vi "RT Loop - Analyze Acceleration_2.vi"(7 "testing":bool, 8 "error in (no error)":errorcluster, 9 "Acceleration RT FIFO In":T1, 10 "FPGA VI Reference Out":refnum<k20>, 11 "Message Queue":refnum<queue>) -> (1 "Acceleration RT FIFO Out":T1)   [LabVIEW 2017]
doc: "Read and analyze acceleration waveform data from FPGA via DMA FIFO. If the acceleration is over the limit, then send the acceleration waveform data to the Log Data Loop."
uses:
  UI Error Handlers/support/Message Queue/Message Cluster.ctl
  controls/Acceleration RT FIFO Reference.ctl
  Globals/Global - All RT Loop Stop.vi
  Globals/Global - Configuration Options.vi
  <vilib>/Utility/error.llb/Error Cluster From Error Code.vi
  <vilib>/rvi/errors/niLvFpgaAdjustHostInterfaceError.vi
  <vilib>/rvi/interface/nirviMethod/nirviMethod.xnode
  <vilib>/FPGAPlugInAG/Dynamic/niLvFpga_ReadFifo_Dynamic.vi
  <vilib>/rvi/errors/niLvFpgaMergeErrorWithErrorCode.vi
  UI Error Handlers/support/Logging/Logging.lvlib
  UI Error Handlers/support/Message Queue/Message Queue.lvlib
panel:
  out "G1 status":cluster{"G1 trigger":bool}
  out "G1 status.G1 trigger":bool
  out "sta":bool
  out "logical OR":bool
  in  "Data Rate (Hz)":dbl
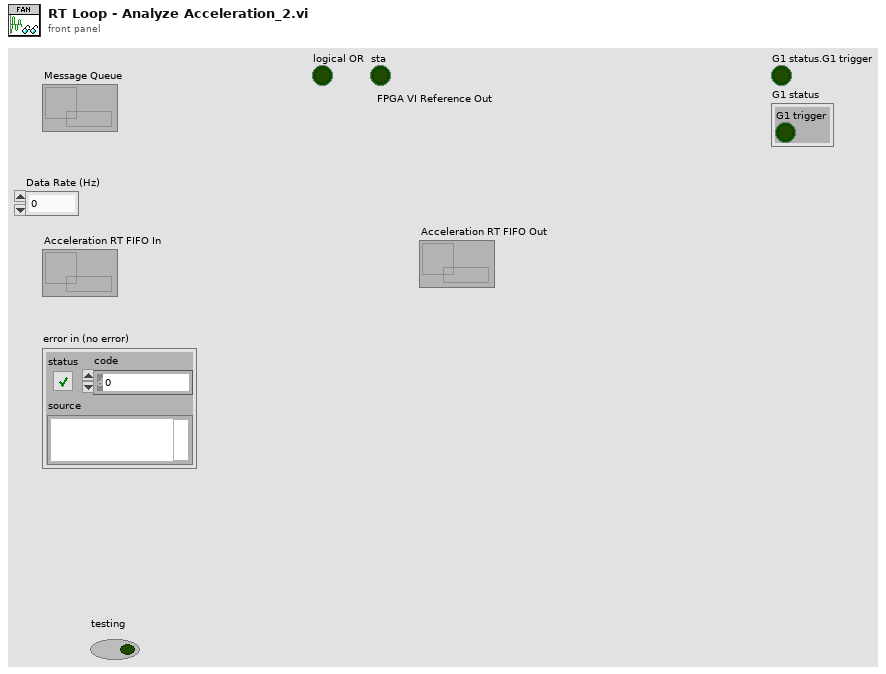
[diagram p1: front panel]
types:
  T1 = typedef "Acceleration RT FIFO Reference.ctl" = refnum<k33>
  T2 = cluster{"Tool data":cluster{"Number of teeth":sgl}, "Cutting data":cluster{"rpm":sgl}, "Limits":cluster{"Magnitude threshold":sgl, "Tolerance":sgl}, "G1 status":cluster{"G1 trigger":bool}}
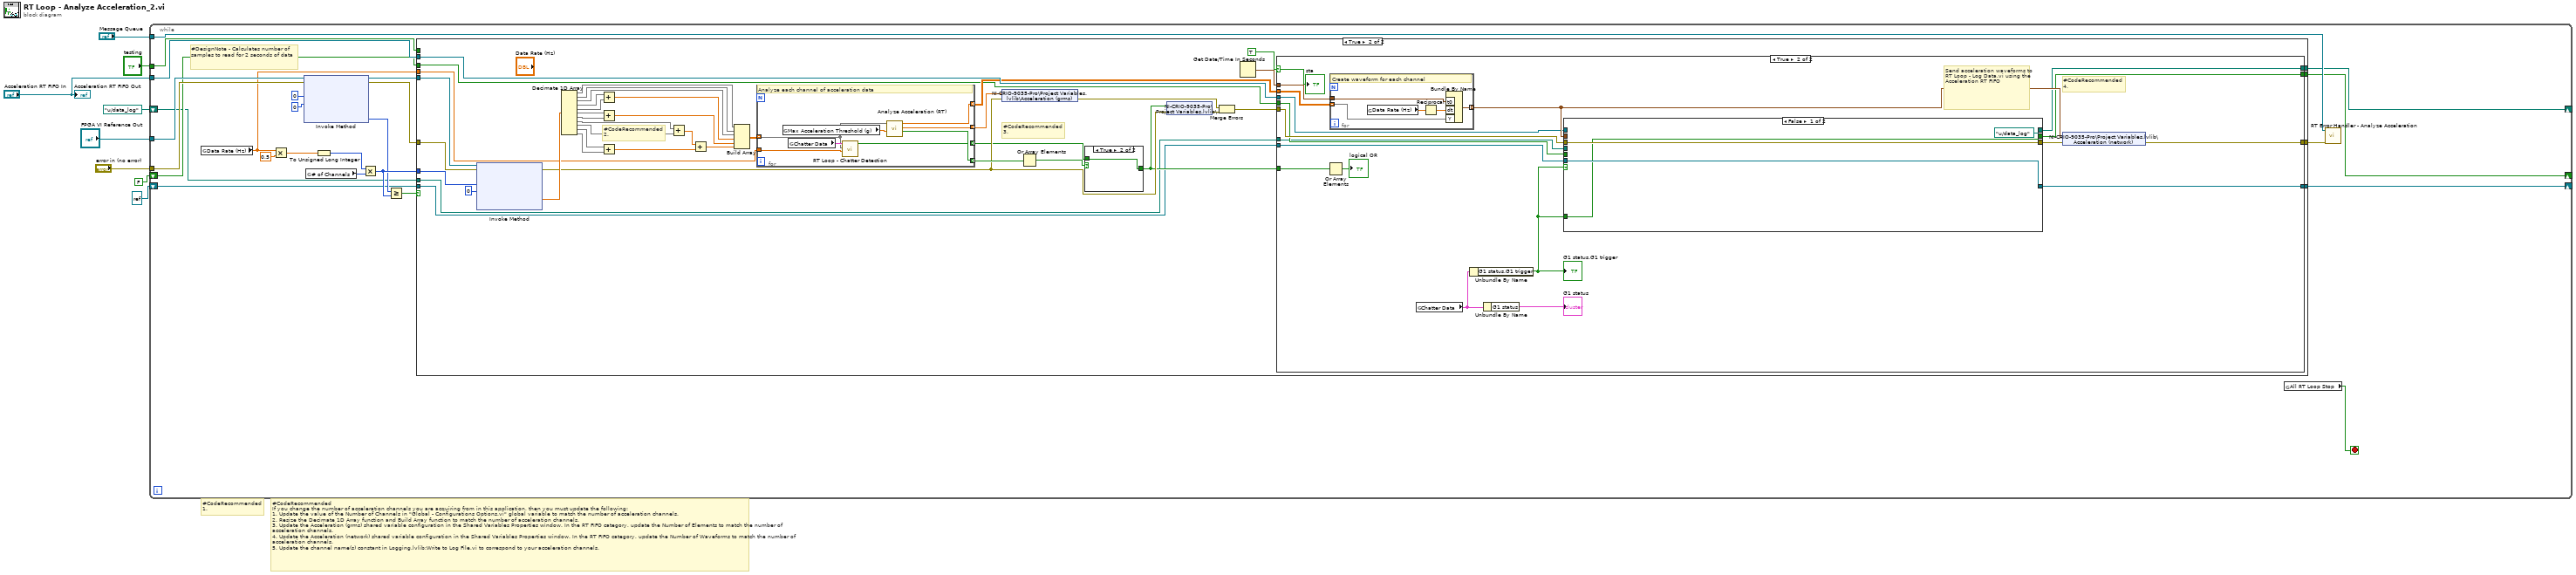
[diagram p0: block diagram]
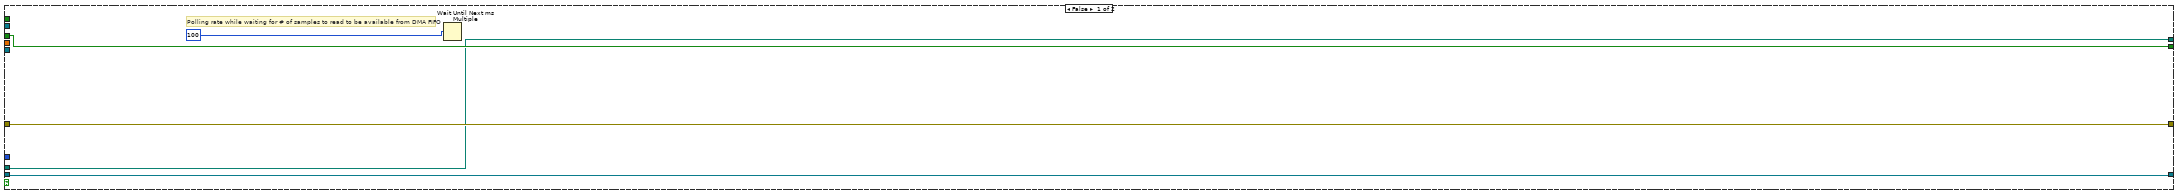
[diagram p2: hidden frame]
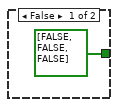
[diagram p3: hidden frame]
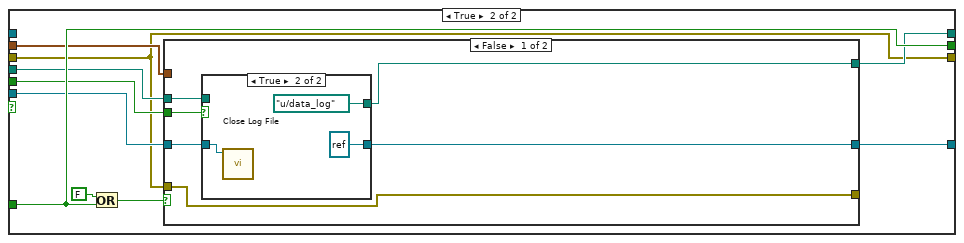
[diagram p5: hidden frame]
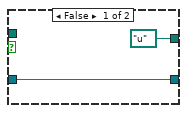
[diagram p6: hidden frame]
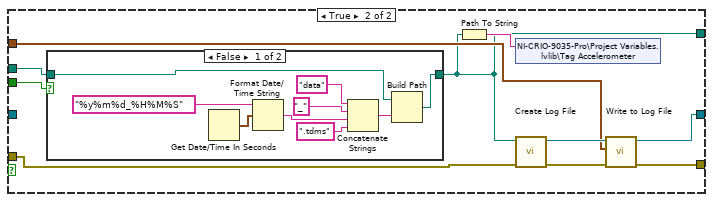
[diagram p7: hidden frame]
diagram:
  # "#CodeRecommended\n1."
  # "#CodeRecommended\nIf you change the number of acceleration channels you are acquiring from in this application, then you must update the following:\n1. Update the value of the Number of Channels in \"Global - Configurations Options.vi\" global variable to match the number of acceleration channels.\n2. Resize the Decimate 1D Array function and Build Array function to match the number of acceleration channels. \n3. Update the Acceleration (grms) shared variable configuration in the Shared Variables Properties window. In the RT FIFO category, update the Number of Elements to match the number of acceleration channels. \n4. Update the Acceleration (network) shared variable configuration in the Shared Variables Properties window. In the RT FIFO category, update the Number of Waveforms to match the number of acceleration channels.\n5. Update the channel name(s) constant in Logging.lvlib:Write to Log File.vi to correspond to your acceleration channels."
  n1 = while {
    tunnel: "FPGA VI Reference Out" -> [w33]
    tunnel: "error in (no error)" -> [w32]
    tunnel: "Message Queue" -> [w25]
    tunnel: "Acceleration RT FIFO In" -> [w23]
    tunnel: "testing" -> [w15]
    shift-right: [w12] -> _
    shift-left: path "u:/data_log" ("AVI Path") -> [w11]
    shift-right: [w14] -> _
    shift-left: FALSE -> [w13]
    shift-right: [w10] -> _
    shift-left: refnum<k34> refnum ("Log File out") -> [w9]
    stop <- w26 stop-if-true
    # "#DesignNote - Calculates number of samples to read for 2 seconds of data"
    n2 = global read "Global - Configuration Options.vi" "Data Rate (Hz)"() -> (w17:dbl)
    n3 = Multiply(x=w17, y=0.5) -> (x*y=w21:dbl)
    n4 = xnode "Invoke Method"("FPGA VI Reference In"=w33, "error in"=w32, "Number of Elements"=u32 0, "Timeout (ms)"=0) -> ("FPGA VI Reference Out"=w29:refnum<k20>, "error out"=w28:errorcluster, "Elements Remaining"=w16:u32)  [unwired: 1 out]
    n5 = global read "Global - Configuration Options.vi" "# of Channels"() -> (w18:u32)
    n6 = To Unsigned Long Integer(number=w21) -> (unsigned 32bit integer=w20:u32)
    n7 = Multiply(x=w20, y=w18) -> (x*y=w19:u32)
    n8 = Greater Or Equal?(x=w16, y=w19) -> (x >= y?=w27:bool)
    n9 = case shown="True" w27 {
      tunnel: w29 -> [_ w81]
      tunnel: w28 -> [w38 w80]
      tunnel: [w38 w76] -> w24
      tunnel: w19 -> [_ w79]
      tunnel: w23 -> [_ w74]
      tunnel: w17 -> [_ w70]
      tunnel: w15 -> [_ _]
      tunnel: [w36 w62] -> w14
      tunnel: w13 -> [w36 w61]
      tunnel: [w35 w60] -> w12
      tunnel: w11 -> [w35 w59]
      tunnel: [w34 w58] -> w10
      tunnel: w9 -> [w34 w57]
      frame False {
        # "Polling rate while waiting for # of samples to read to be available from DMA FIFO"
        n10 = Wait Until Next ms Multiple(millisecond multiple=u32 100) -> ()  [unwired: 1 out]
      }
      frame True {
        # "#CodeRecommended\n3."
        # "#CodeRecommended\n2."
        n11 = xnode "Invoke Method"("FPGA VI Reference In"=w81, "error in"=w80, "Number of Elements"=w79, "Timeout (ms)"=0) -> ("error out"=w69:errorcluster, "Data"=w73:sgl[])  [unwired: 2 out]
        n12 = Decimate 1D Array(w73) -> (w54:sgl[], w53:sgl[], w52:sgl[], w51:sgl[], w50:sgl[], w48:sgl[], w47:sgl[], w46:sgl[], w45:sgl[], w44:sgl[], w43:sgl[])
        n13 = Add(x=w51, y=w50) -> (x+y=w49:sgl[])
        n14 = Add(x=w48, y=w47) -> (x+y=w39:sgl[])
        n15 = Add(x=w44, y=w43) -> (x+y=w41:sgl[])
        n16 = Add(x=w46, y=w45) -> (x+y=w42:sgl[])
        n17 = Add(x=w42, y=w41) -> (x+y=w40:sgl[])
        n18 = Build Array(w54, w53, w52, w49, w39, w40) -> (w55:sgl[][])
        n19 = for {
          tunnel: [w91] -> w75 mode=indexing
          tunnel: [w90] -> w72 mode=indexing
          tunnel: [w89] -> w71 mode=indexing
          tunnel: w70 -> [w87]
          tunnel: [w86] -> w64 mode=indexing
          tunnel: w55 -> [w84] mode=indexing
          # "Analyze each channel of acceleration data"
          n20 = global read "Global - Configuration Options.vi" "Max Acceleration Threshold (g)"() -> (w88:sgl)
          n21 = global read "Global - Configuration Options.vi" "Chatter Data"() -> (w85:T2)
          n22 = call "RT Loop - Chatter Detection.vi"("Data Rate (Hz)"=w87, "Acceleration Waveform (SGL)"=w84, "Chatter Data"=w85) -> ("Chatter?"=w86:bool)  [unwired: 8 in]
          n23 = call "Analyze Acceleration (RT).vi"("Max Instantaneous Acceleration (g)"=w88, "Acceleration Waveform (SGL)"=w84) -> ("Over Limit?"=w91:bool, "Acceleration (grms)"=w89:dbl, "Acceleration Waveform (DBL)"=w90:dbl[])  [unwired: 7 in]
        }
        n24 = shared-variable "NI-CRIO-9035-Pro\\Project Variables.lvlib\\Acceleration (grms)"(w71, error in=w69) -> (error out=w67:errorcluster)
        n25 = Or Array Elements(Boolean array=w75) -> (logical OR=w65:bool)
        n26 = case shown="True" w65 {
          tunnel: w64 -> [_ w83]
          tunnel: [bool[] [FALSE, FALSE, FALSE] ("Chatter?") w83] -> w63
          frame False {
          }
          frame True {
          }
        }
        n27 = shared-variable "NI-CRIO-9035-Pro\\Project Variables.lvlib\\Chatter?"(w63, error in=w69) -> (error out=w68:errorcluster)
        n28 = Merge Errors(w67, w68) -> (w66:errorcluster)
        n29 = Get Date/Time In Seconds() -> (seconds since 1Jan1904=w77:timestamp)
        n30 = case shown="True" TRUE {
          selector: TRUE -> [_ w106]
          tunnel: w77 -> [_ w114]
          tunnel: w66 -> [w95 w113]
          tunnel: [w95 w112] -> w76
          tunnel: w74 -> [_ w110]
          tunnel: w72 -> [_ w109]
          tunnel: w63 -> [_ w107]
          tunnel: [w94 w103] -> w62
          tunnel: w61 -> [w94 w102]
          tunnel: [w93 w101] -> w60
          tunnel: w59 -> [w93 w96]
          tunnel: [w92 w100] -> w58
          tunnel: w57 -> [w92 w99]
          frame False {
          }
          frame True {
            # "#CodeRecommended\n4."
            # "Send acceleration waveforms to RT Loop - Log Data.vi using the Acceleration RT FIFO"
            n31 = Or Array Elements(Boolean array=w107) -> (logical OR=→"logical OR":bool)
            n32 = for {
              tunnel: w109 -> [w164] mode=indexing
              tunnel: w114 -> [w163]
              tunnel: [w161] -> w111 mode=indexing
              # "Create waveform for each channel"
              n33 = global read "Global - Configuration Options.vi" "Data Rate (Hz)"() -> (w160:dbl)
              n34 = Reciprocal(x=w160) -> (1/x=w162:dbl)
              n35 = Bundle By Name("t0"=w163, "dt"=w162, "Y"=w164) -> (w161:waveform(dbl))  [unwired: 1 in]
            }
            n36 = global read "Global - Configuration Options.vi" "Chatter Data"() -> (w105:T2)
            n37 = Unbundle By Name(w105) -> ("G1 status.G1 trigger"=w97:bool)
            "G1 status.G1 trigger" <- w97
            n38 = Unbundle By Name(w105) -> ("G1 status"=→"G1 status":cluster{"G1 trigger":bool})
            n39 = case shown="False" w97 {
              tunnel: w113 -> [w118 w119]
              tunnel: w111 -> [_ w120]
              tunnel: w110 -> [_ _]
              tunnel: w97 -> [w116 w126]
              tunnel: [w116 w126] -> w103
              tunnel: w102 -> [_ w125]
              tunnel: [path "u:/data_log" ("AVI Path") w124] -> w101
              tunnel: w96 -> [_ w123]
              tunnel: [w117 w122] -> w100
              tunnel: w99 -> [w117 w121]
              tunnel: [w118 w119] -> w98
              frame False {
              }
              frame True {
                n40 = Or(x=FALSE, y=w126) -> (x .or. y?=w128:bool)
                n41 = case shown="False" w128 {
                  tunnel: w123 -> [w131 w149]
                  tunnel: [w134 w143] -> w124
                  tunnel: w125 -> [w132 w148]
                  tunnel: w121 -> [w133 _]
                  tunnel: w120 -> [_ w145]
                  tunnel: [w130 w142] -> w122
                  tunnel: w119 -> [w129 w141]
                  tunnel: [w129 w140] -> _
                  frame False {
                    n42 = case shown="True" w132 {
                      tunnel: [path "u:/" ("AVI Path") path "u:/data_log" ("AVI Path")] -> w134
                      tunnel: w133 -> [w135 w138]
                      tunnel: w131 -> [_ _]
                      tunnel: [w135 refnum<k34> refnum ("Log File out")] -> w130
                      frame False {
                      }
                      frame True {
                        n43 = call "Close Log File.vi"("tdms file"=w138) -> ()  [unwired: 10 in, 1 out]
                      }
                    }
                  }
                  frame True {
                    n44 = case shown="False" w148 {
                      tunnel: w149 -> [w151 w159]
                      tunnel: [w150 w159] -> w143
                      frame False {
                        n45 = Get Date/Time In Seconds() -> (seconds since 1Jan1904=w154:timestamp)
                        n46 = Format Date/Time String(time format string (%c)="%y%m%d_%H%M%S", seconds (now)=w154) -> (date/time string=w157:string)  [unwired: 1 out]
                        n47 = Concatenate Strings("data" ("string"), "_" ("string"), w157, ".tdms" ("string")) -> (w152:string)
                        n48 = Build Path(base path=w151, name or relative path=w152) -> (appended path=w150:path)
                      }
                      frame True {
                      }
                    }
                    n49 = Path To String(path=w143) -> (string=w144:string)
                    n50 = shared-variable "NI-CRIO-9035-Pro\\Project Variables.lvlib\\Tag Accelerometer"(w144) -> ()  [unwired: 1 in, 1 out]
                    n51 = call "Create Log File.vi"("error in (no error)"=w141, "Acceleration Exceeded Log Folder"=w143) -> ("error out"=w147:errorcluster, "Log File out"=w146:refnum<k34>)  [unwired: 8 in]
                    n52 = call "Write to Log File.vi"("error in (no error)"=w147, "Array of Waveforms"=w145, "Log File in"=w146) -> ("error out"=w140:errorcluster, "Log File out"=w142:refnum<k34>)  [unwired: 7 in]
                  }
                }
              }
            }
            n53 = shared-variable "NI-CRIO-9035-Pro\\Project Variables.lvlib\\Acceleration (network)"(w111, error in=w98) -> (error out=w112:errorcluster)
            "sta" <- w106
          }
        }
      }
    }
    n54 = global read "Global - All RT Loop Stop.vi" "All RT Loop Stop"() -> (w26:bool)
    n55 = call "RT Error Handler - Analyze Acceleration.vi"("error in (no error)"=w24, "Message Queue"=w25) -> ()  [unwired: 9 in, 1 out]
  }
  "Acceleration RT FIFO Out" <- "Acceleration RT FIFO In"
